vi "commandEnable.vi"(8 "error in (no error)":errorcluster, 10 "CommandEnable in":T1, 11 "Communicator in":refnum<class "Communicator.lvclass">) -> (0 "error out":errorcluster, 2 "CommandEnable out":T1, 3 "Communicator out":refnum<class "Communicator.lvclass">)   [LabVIEW 2016, in "M1M3Communicator.lvlib" / "Communicator.lvclass"]
uses:
  Communicator.lvclass
  Topics/CommandEnable.ctl
  Topics/CommandId.ctl
  M1M3Communicator.lvlib
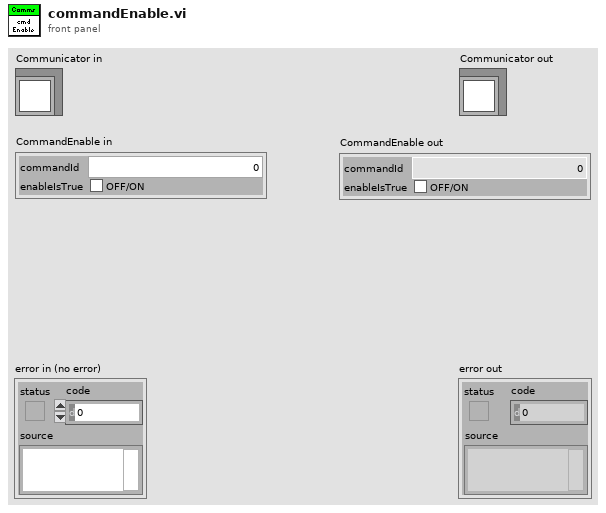
[diagram p1: front panel]
types:
  T1 = typedef "M1M3Communicator.lvlib/CommandEnable.ctl" = cluster{"commandId":T2, "enableIsTrue":bool}
  T2 = typedef "M1M3Communicator.lvlib/CommandId.ctl" = i32
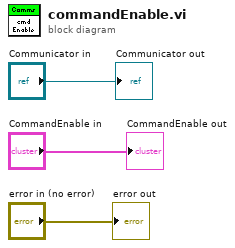
[diagram p0: block diagram]
diagram:
  "error out" <- "error in (no error)"
  "Communicator out" <- "Communicator in"
  "CommandEnable out" <- "CommandEnable in"
